vi "Get Node Ref.vi"(8 "error in (no error)":errorcluster, 10 "XPath expression":string, 11 "Project XML Editor in":refnum<class "Project XML Editor.lvclass">) -> (0 "error out":errorcluster, 1 "Found?":bool, 2 "Node ref out":refnum<k20>, 3 "Project XML Editor out":refnum<class "Project XML Editor.lvclass">)   [LabVIEW 2020, in "LVLIBP CD XML Updater.lvlib" / "Project XML Editor.lvclass"]
uses:
  Project XML Editor.lvclass
  Project XML Editor.lvclass/Project XML Editor.ctl
  <vilib>/xml/NI_XML.lvlib
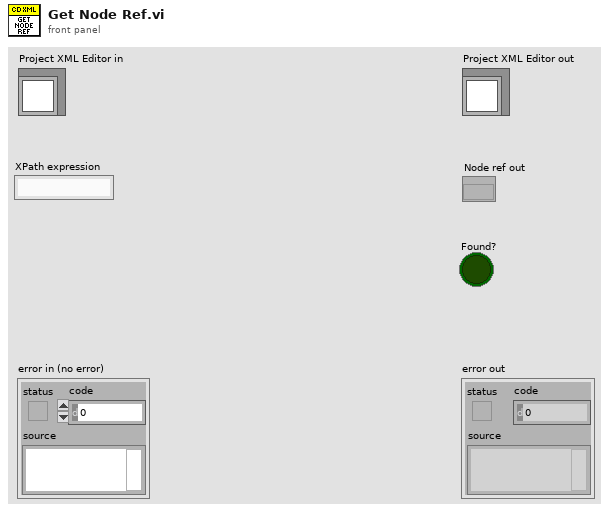
[diagram p1: front panel]
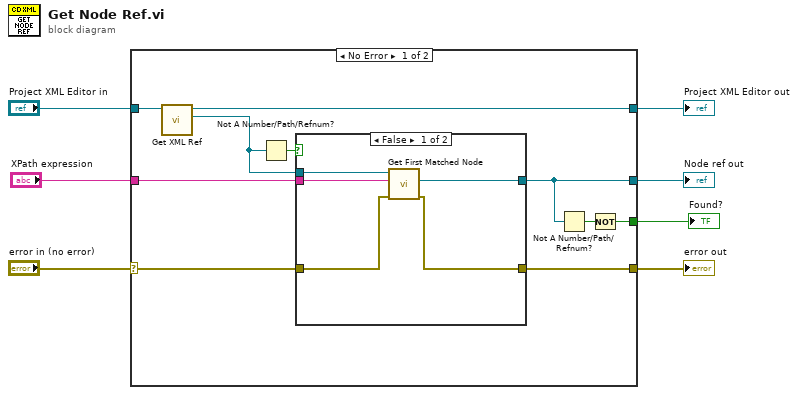
[diagram p0: block diagram]
diagram:
  n1 = case shown="No Error" "error in (no error)" {
    selector: "error in (no error)" -> [w16 w25]
    tunnel: [w13 w25] -> w6
    tunnel: [w12 w24] -> w4
    tunnel: "Project XML Editor in" -> [w17 w24]
    tunnel: [w10 _] -> w3
    tunnel: "XPath expression" -> [w11 _]
    tunnel: [w8 _] -> w1
    frame No Error {
      n2 = call "Get XML Ref.vi"("Project XML Editor in"=w17) -> ("XML Ref"=w14:refnum<k20>, "Project XML Editor out"=w12:refnum<class "Project XML Editor.lvclass">)  [unwired: 9 in]
      n3 = Not A Number/Path/Refnum?(number/path/refnum=w14) -> (NaN/Path/Refnum?=w15:bool)
      n4 = case shown="False" w15 {
        tunnel: w16 -> [w21 w23]
        tunnel: w14 -> [w22 _]
        tunnel: [w20 w23] -> w13
        tunnel: [w19 _] -> w10
        tunnel: w11 -> [w18 _]
        frame False {
          n5 = call <vilib>:"Get First Matched Node.vi"("error in (no error)"=w21, "XPath expression"=w18, "node in"=w22) -> ("error out"=w20:errorcluster, "node result"=w19:refnum<k20>)  [unwired: 6 in, 1 out]
        }
        frame True {
        }
      }
      n6 = Not A Number/Path/Refnum?(number/path/refnum=w10) -> (NaN/Path/Refnum?=w9:bool)
      n7 = Not(x=w9) -> (.not. x?=w8:bool)
    }
    frame Error {
    }
  }
  "error out" <- w6
  "Project XML Editor out" <- w4
  "Node ref out" <- w3
  "Found?" <- w1
